vi "3D_Mesh_Plot_Merge_VI.vi"() -> ()   [LabVIEW 2020]
uses:
  <vilib>/Math Plots/3D Math Plots/3D Mesh/3D Mesh XCtrl/3D Mesh.xctl
  <vilib>/Math Plots/3D Math Plots/3D Mesh/3D Mesh Datatype/Public/Plot Helper (Matrix).vi
  <vilib>/Math Plots/3D Math Plots/3D Mesh/3D Mesh Datatype/3D Mesh Datatype.lvclass
panel:
  out "3D Mesh":refnum<class "3D Plot Datatype.lvclass">[](xcontrol)
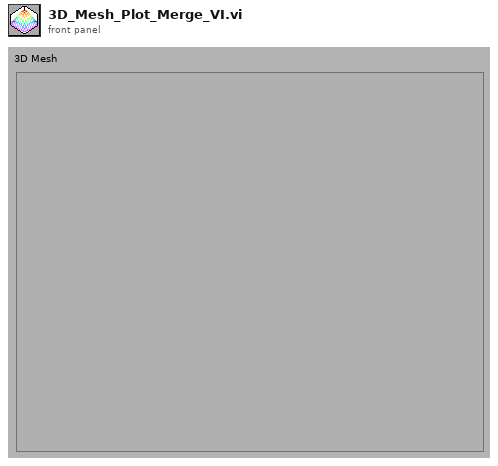
[diagram p1: front panel]
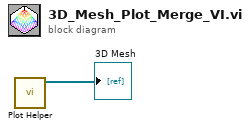
[diagram p0: block diagram]
diagram:
  n1 = call-poly <vilib>:"Plot Helper.vi"() -> ("3D Plot lvclass Array out"=→"3D Mesh":refnum<class "3D Plot Datatype.lvclass">[])  [unwired: 6 in, 5 out]
